vi "Set Events.vi"(8 "error in (no error)":errorcluster, 10 "Events":cluster{"Event Log Entry":refnum<user-event>}, 11 "Series UI Actor in":refnum<class "Series UI Actor.lvclass">) -> (0 "error out":errorcluster, 3 "Series UI Actor out":refnum<class "Series UI Actor.lvclass">)   [LabVIEW 2024, in "Series UI Actor.lvlib" / "Series UI Actor.lvclass"]
uses:
  Series UI Actor.lvclass
  Series UI Actor.lvclass/Series UI Actor.ctl
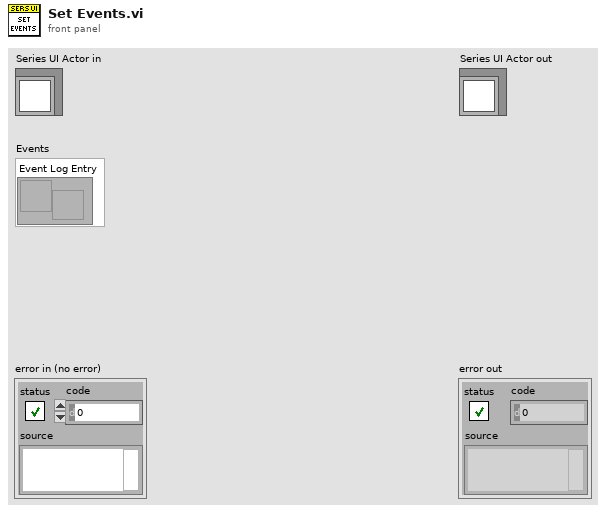
[diagram p1: front panel]
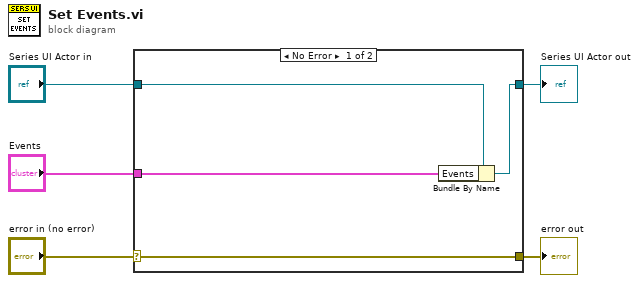
[diagram p0: block diagram]
diagram:
  n1 = case shown="No Error" "error in (no error)" {
    selector: "error in (no error)" -> [w9 w10]
    tunnel: [w9 w10] -> w4
    tunnel: [w7 w11] -> w2
    tunnel: "Series UI Actor in" -> [w8 w11]
    tunnel: "Events" -> [w6 _]
    frame No Error {
      n2 = Bundle By Name(cluster=w8, "Events"=w6) -> (w7:refnum<class "Series UI Actor.lvclass">)
    }
    frame Error {
    }
  }
  "error out" <- w4
  "Series UI Actor out" <- w2
